vi "Shutdown.vi"(7 "LabVIEW Web Service Request":refnum<class "Web Request.lvclass">) -> ()   [LabVIEW 2017]
uses:
  <vilib>/wsapi/Web Request.lvclass
  Controller/Messages/Send Shutdown MSG/Send Shutdown MSG.lvclass
  C:/Program Files (x86)/National Instruments/LabVIEW 2017/vi.lib/ActorFramework/Message/Message.lvclass
  <vilib>/ActorFramework/Message Enqueuer/Message Enqueuer.lvclass/Message Enqueuer.ctl
  <vilib>/ActorFramework/Message Priority Queue/Priority Enqueue.vi
  Controller/gController.lvclass
  <vilib>/ActorFramework/Message Enqueuer/Message Enqueuer.lvclass
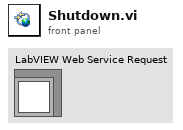
[diagram p1: front panel]
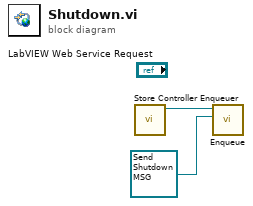
[diagram p0: block diagram]
diagram:
  n1 = call "Store Controller Enqueuer.vi"() -> ("Controller Enqueuer Out"=w2:refnum<class "Message Enqueuer.lvclass">)  [unwired: 11 in]
  n2 = call <vilib>:"Enqueue.vi"("Message"=refnum<class "Send Shutdown MSG.lvclass"> refnum ("Controller.lvlib:Send Shutdown MSG.lvclass"), "Message Enqueuer in"=w2) -> ()  [unwired: 8 in, 2 out]
